vi "Demo.vi"() -> ()   [LabVIEW 2011, in "Gif Image.lvclass"]
uses:
  Gif Class/Gif Image.lvclass
  Gif Class/Control/Application Extension.ctl
  Gif Class/Control/ID Charactor.ctl
panel:
  out "无符号字节数组":u8[](array[numeric]) format="%.0x"
  out "Gif data":string
  out "Offset":i32
  out "子字符串":string
  out "Application Extension":T1 {"Application Extension Labe(1)l" format="0x%02x" items=["Image Seperator"=44, "Extension Introducer"=33, "Graphic Control Label"=249, "Comment Label"=254, "PlainText Label"=1, "Gif Trailor"=59, "Application Label"=255]; "ID(1)" format="0x%02x" items=["Image Seperator"=44, "Extension Introducer"=33, "Graphic Control Label"=249, "Comment Label"=254, "PlainText Label"=1, "Gif Trailor"=59, "Application Label"=255]}
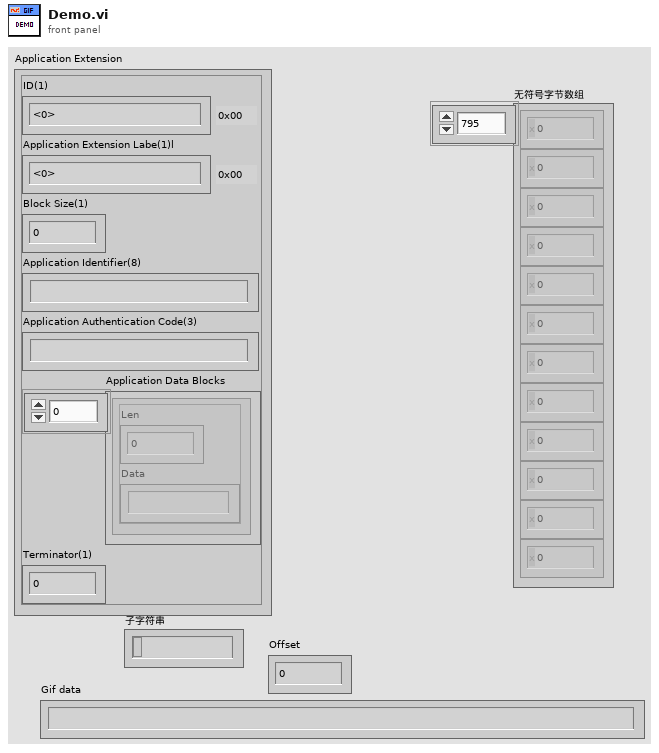
[diagram p1: front panel]
types:
  T1 = typedef "Gif Image.lvclass/Application Extension.ctl" = cluster{"ID(1)":T2, "Application Extension Labe(1)l":T2, "Block Size(1)":u8, "Application Identifier(8)":string, "Application Authentication Code(3)":string, "Application Data Blocks":cluster{"Len":u8, "Data":string}[], "Terminator(1)":u8}
  T2 = typedef "Gif Image.lvclass/ID Charactor.ctl" = u8
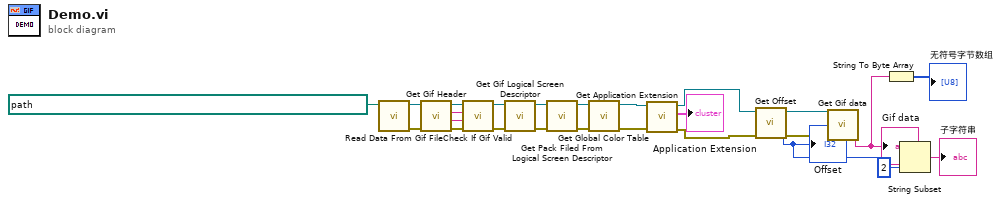
[diagram p0: block diagram]
diagram:
  n1 = call "Read Data From Gif File.vi"("Gif File Path"=path "E:/BOOK/功能块/图片工具/Image File/gif/demo gif/demo.gif") -> ("Gif Image 输出"=w24:refnum<class "Gif Image.lvclass">, "error out"=w23:errorcluster)  [unwired: 8 in]
  n2 = call "Get Gif Header.vi"("error in (no error)"=w23, "Gif Image 输入"=w24) -> ("error out"=w19:errorcluster, "Version"=w20:string, "Signature"=w21:string, "Gif Image 输出"=w22:refnum<class "Gif Image.lvclass">)  [unwired: 6 in]
  n3 = call "Check If Gif Valid.vi"("error in (no error)"=w19, "Version"=w20, "Signature"=w21, "Gif Image 输入"=w22) -> ("error out"=w18:errorcluster, "Gif Image 输出"=w17:refnum<class "Gif Image.lvclass">)  [unwired: 5 in, 1 out]
  n4 = call "Get Gif Logical Screen Descriptor.vi"("error in (no error)"=w18, "Gif Image 输入"=w17) -> ("error out"=w15:errorcluster, "Gif Image 输出"=w16:refnum<class "Gif Image.lvclass">)  [unwired: 8 in]
  n5 = call "Get Pack Filed From Logical Screen Descriptor.vi"("error in (no error)"=w15, "Gif Image 输入"=w16) -> ("error out"=w13:errorcluster, "Gif Image 输出"=w14:refnum<class "Gif Image.lvclass">)  [unwired: 8 in]
  n6 = call "Get Global Color Table.vi"("error in (no error)"=w13, "Gif Image 输入"=w14) -> ("error out"=w11:errorcluster, "Gif Image 输出"=w12:refnum<class "Gif Image.lvclass">)  [unwired: 8 in]
  n7 = call "Get Application Extension.vi"("error in (no error)"=w11, "Gif Image 输入"=w12) -> ("error out"=w8:errorcluster, "Application Extension"=→"Application Extension":T1, "Gif Image 输出"=w9:refnum<class "Gif Image.lvclass">)  [unwired: 7 in]
  n8 = call "Get Offset.vi"("error in (no error)"=w8, "Gif Image输入"=w9) -> ("error out"=w6:errorcluster, "Offset"=w5:i32, "Gif Image输出"=w7:refnum<class "Gif Image.lvclass">)  [unwired: 7 in]
  "Offset" <- w5
  n9 = call "Get Gif data.vi"("error in (no error)"=w6, "Gif Image输入"=w7) -> ("Gif data"=w2:string)  [unwired: 7 in, 2 out]
  "Gif data" <- w2
  n10 = String To Byte Array(string=w2) -> (unsigned byte array=→"无符号字节数组":u8[])
  n11 = String Subset(string=w2, offset (0)=w5, length (rest)=2 ("长度（剩余）")) -> (substring=→"子字符串":string)
